vi "VGF.vi"(7 "Enum":enum16{"GET VALUE", "SET VALUE", "RESET"}(ring), 9 "STOP":bool) -> (1 "OUT":bool)   [LabVIEW 2014]
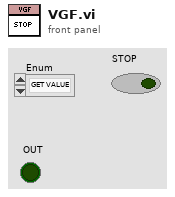
[diagram p1: front panel]
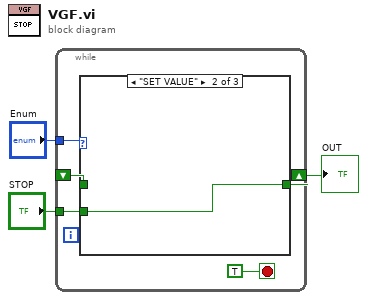
[diagram p0: block diagram]
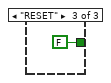
[diagram p3: hidden frame]
diagram:
  n1 = while {
    shift-right: [w6] -> w2
    shift-left: _ -> [w4]
    tunnel: "Enum" -> [w7]
    tunnel: "STOP" -> [w5]
    stop <- TRUE stop-if-true
    n2 = case shown="\"SET VALUE\"" w7 {
      tunnel: [w9 w10 FALSE ("STOP")] -> w6
      tunnel: w5 -> [_ w10 _]
      tunnel: w4 -> [w9 _ _]
      frame "GET VALUE", Default {
      }
      frame "SET VALUE" {
      }
      frame "RESET" {
      }
    }
  }
  "OUT" <- w2
